vi "Apply-gaussian-filter.vi"(8 "error in":errorcluster, 9 "Corrected":T1[](array[typedef]), 10 "Kernel Number":i32=4, 11 "Kernel Size":i32=3) -> (0 "error IO":errorcluster)   [LabVIEW 2013, in "CameraVision.lvlib" / "CV-Correction.lvclass"]
uses:
  CV-Correction.lvclass
  <vilib>/vision/Image Controls.llb/IMAQ Image.ctl
  <vilib>/vision/NI_Vision_Development_Module.lvlib
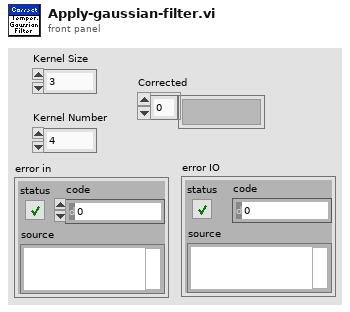
[diagram p1: front panel]
types:
  T1 = typedef "IMAQ Image.ctl" = refnum<image>
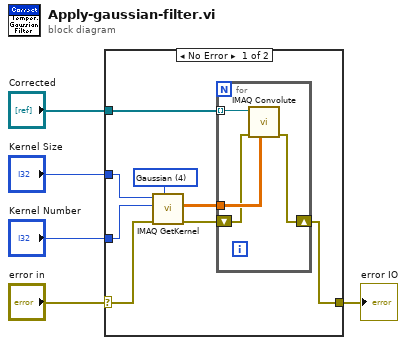
[diagram p0: block diagram]
diagram:
  n1 = case shown="No Error" "error in" {
    selector: "error in" -> [w12 w18]
    tunnel: [w13 w18] -> w5
    tunnel: "Kernel Size" -> [w8 _]
    tunnel: "Kernel Number" -> [w7 _]
    tunnel: "Corrected" -> [w6 _]
    frame No Error {
      w11 = u16 4 items=["Gradient"=1, "Laplacian"=2, "Smoothing"=3, "Gaussian"=4] ("Kernel Family")
      n2 = call "IMAQ GetKernel"("Kernel Family"=w11, "error in (no error)"=w12, "Kernel Number"=w7, "Kernel Size (3,5,...)"=w8) -> ("error out"=w9:errorcluster, "Kernel"=w10:sgl[][])  [unwired: 4 in, 2 out]
      n3 = for {
        tunnel: w10 -> [w16]
        tunnel: w6 -> [w14] mode=indexing
        shift-right: [w17] -> w13
        shift-left: w9 -> [w15]
        n4 = call "IMAQ Convolute"("Kernel"=w16, "error in (no error)"=w15, "Image Src"=w14) -> ("error out"=w17:errorcluster)  [unwired: 7 in, 1 out]
      }
    }
    frame Error {
    }
  }
  "error IO" <- w5
